vi "monochromatorInitialize.vi"(8 "error in":errorcluster, 9 "command_wait_time":i32, 10 "dev_timeout":u32, 11 "monochromator":refnum<k24>) -> (0 "error out":errorcluster, 3 "reference out":refnum<k24>)   [LabVIEW 2009]
doc: "Initalize Monochromator\nSet Device Connection (Bulk In/Out) Timeout (500ms)\nSet Command Wait Time (100ms)\n\nIf default values are used this VI is not required to initialize the device"
uses:
  C:/Users/anderson.chen/Desktop/Software Development/Cornerstone Series API (LV9)/Cornerstone DLL/Cornerstone.dll
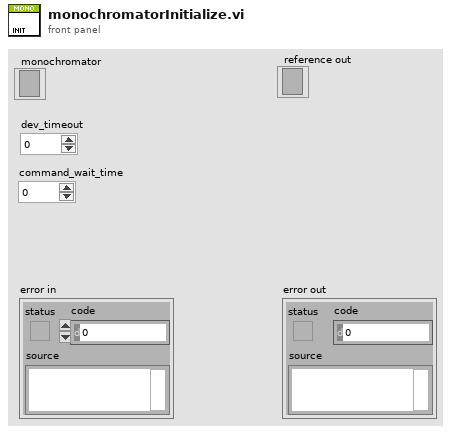
[diagram p1: front panel]
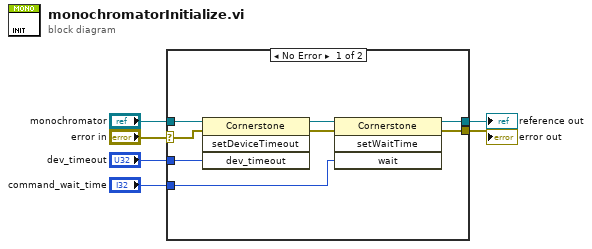
[diagram p0: block diagram]
diagram:
  n1 = case shown="No Error" "error in" {
    selector: "error in" -> [w8 w15]
    tunnel: "monochromator" -> [w14 w16]
    tunnel: "dev_timeout" -> [w13 _]
    tunnel: "command_wait_time" -> [w11 _]
    tunnel: [w10 w16] -> w3
    tunnel: [w9 w15] -> w2
    frame #0 {
      n2 = invoke class="Cornerstone" method="setDeviceTimeout"(reference=w14, error in=w8, "dev_timeout"=w13) -> (reference out=w12:refnum<k24>, error out=w7:errorcluster)  [unwired: 1 in, 2 out]
      n3 = invoke class="Cornerstone" method="setWaitTime"(reference=w12, error in=w7, "wait"=w11) -> (reference out=w10:refnum<k24>, error out=w9:errorcluster)  [unwired: 1 in, 2 out]
    }
    frame #1 {
    }
  }
  "reference out" <- w3
  "error out" <- w2
